vi "Generate Command String.vi"(0 "ITX Commands in":refnum<class "ITX Commands.lvclass">, 3 "error in (no error)":errorcluster) -> (7 "ITX Commands out":refnum<class "ITX Commands.lvclass">, 8 "ITX Commands":string, 10 "error out":errorcluster)   [LabVIEW 2019, in "ITX Commands.lvclass"]
uses:
  ITX Commands.lvclass
  ITX Commands.lvclass/ITX Commands.ctl
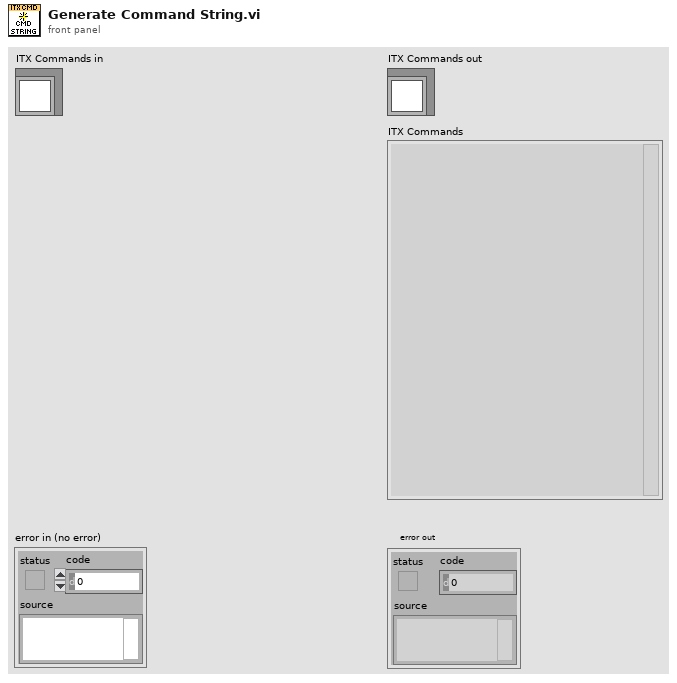
[diagram p1: front panel]
types:
  T1 = cluster{"axThick":string, "grid":string, "height":string, "Log":string, "mirror":string, "prescaleExp":string, "rgb":string, "width":string}
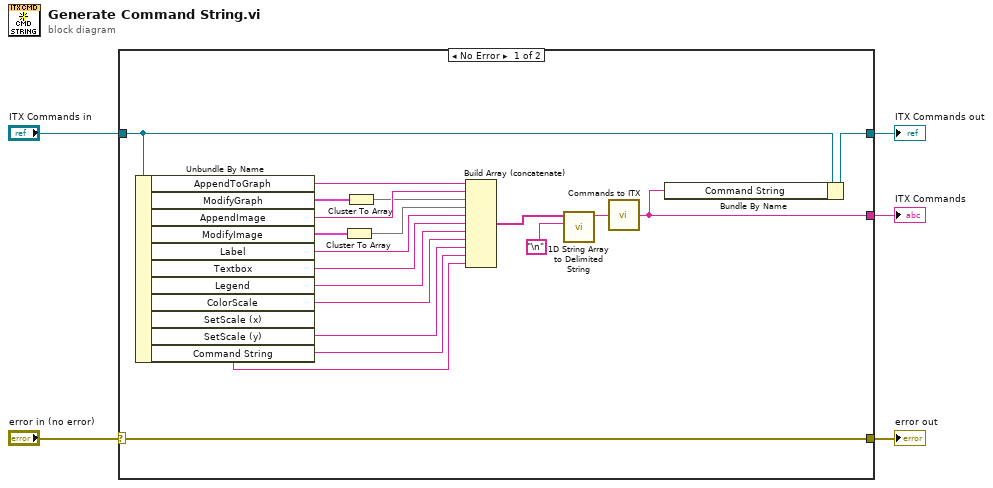
[diagram p0: block diagram]
diagram:
  n1 = case shown="No Error" "error in (no error)" {
    selector: "error in (no error)" -> [w25 w27]
    tunnel: [w25 w27] -> w4
    tunnel: [w8 w26] -> w2
    tunnel: "ITX Commands in" -> [w7 w26]
    tunnel: [w6 _] -> w1
    frame No Error {
      n2 = Unbundle By Name(w7) -> ("AppendToGraph"=w22:string, "ModifyGraph"=w24:T1, "AppendImage"=w16:string, "ModifyImage"=w23:cluster{"ctab":string}, "Label"=w20:string, "Textbox"=w19:string, "Legend"=w18:string, "ColorScale"=w17:string, "SetScale (x)"=w13:string, "SetScale (y)"=w12:string, "Command String"=w11:string)
      n3 = Cluster To Array(cluster=w23) -> (array=w21:string[])
      n4 = Cluster To Array(cluster=w24) -> (array=w15:string[])
      n5 = Build Array (concatenate)(w22, w16, w15, w21, w20, w19, w18, w17, w13, w12, w11) -> (w10:string[])
      n6 = call <vilib>:"1D String Array to Delimited String.vi"("delimiter"="\n", "string array"=w10) -> ("delimited string"=w14:string)  [unwired: 9 in]
      n7 = call "Commands to ITX.vi"("Commands"=w14) -> ("ITX Commands"=w6:string)
      n8 = Bundle By Name(cluster=w7, "Command String"=w6) -> (w8:refnum<class "ITX Commands.lvclass">)
    }
    frame Error {
    }
  }
  "error out" <- w4
  "ITX Commands out" <- w2
  "ITX Commands" <- w1
